vi "Dispense FN - ON - State Status (SubVI).vi"(0 "Values IN":T1 {"Drain Time (s)" format="%.2f"; "Drain Rate (g/sec)" format="%.2f"}, 7 "Min Spray Complete?":bool, 8 "Spray Count":i32, 9 "Measure Delay Complete?":bool, 11 "Max Spray Complete?":bool) -> (15 "Dispense Timeout?":bool, 17 "Complete":bool, 19 "OFF Signal":bool)   [LabVIEW 2009]
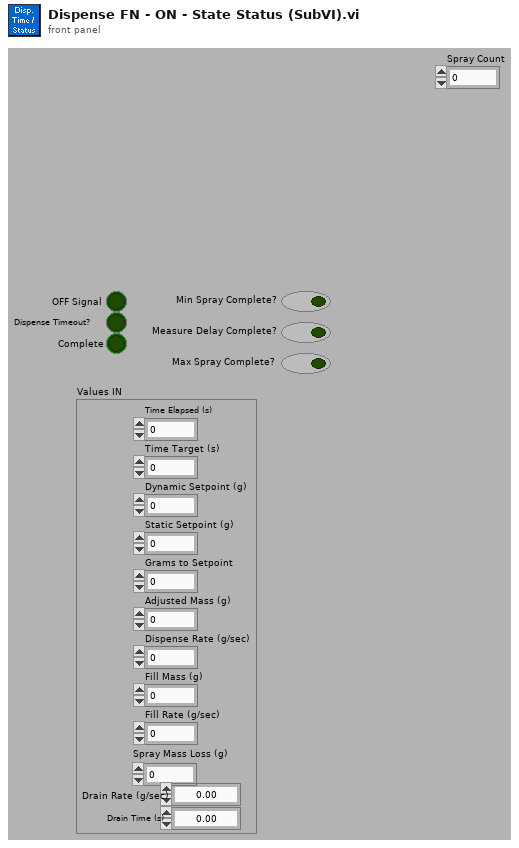
[diagram p1: front panel]
types:
  T1 = cluster{"Time Elapsed (s)":dbl, "Time Target (s)":dbl, "Dynamic Setpoint (g)":dbl, "Static Setpoint (g)":dbl, "Grams to Setpoint":dbl, "Adjusted Mass (g)":dbl, "Dispense Rate (g/sec)":dbl, "Fill Mass (g)":dbl, "Fill Rate (g/sec)":dbl, "Spray Mass Loss (g)":dbl, "Drain Rate (g/sec)":dbl, "Drain Time (s)":dbl}
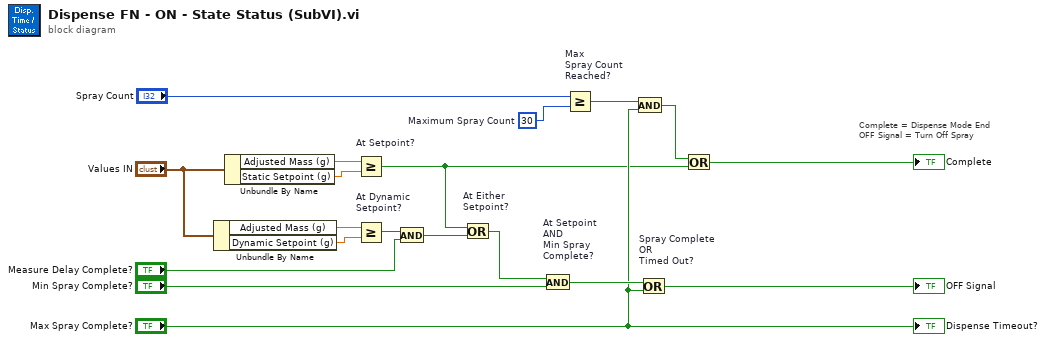
[diagram p0: block diagram]
diagram:
  w7 = 30  # Maximum Spray Count
  # "Complete = Dispense Mode End\nOFF Signal = Turn Off Spray"
  n1 = Unbundle By Name("Values IN") -> ("Adjusted Mass (g)"=w14:dbl, "Dynamic Setpoint (g)"=w15:dbl)
  n2 = Unbundle By Name("Values IN") -> ("Adjusted Mass (g)"=w18:dbl, "Static Setpoint (g)"=w17:dbl)
  n3 = Greater Or Equal? "At Setpoint?"(x=w18, y=w17) -> (x >= y?=w2:bool)
  n4 = Greater Or Equal? "At Dynamic\nSetpoint?"(x=w14, y=w15) -> (x >= y?=w19:bool)
  n5 = And(x=w19, y="Measure Delay Complete?") -> (x .and. y?=w11:bool)
  n6 = Or "At Either\nSetpoint?"(x=w2, y=w11) -> (x .or. y?=w10:bool)
  n7 = And "At Setpoint\nAND\nMin Spray\nComplete?"(x=w10, y="Min Spray Complete?") -> (x .and. y?=w9:bool)
  n8 = Greater Or Equal? "Max\nSpray Count\nReached?"(x="Spray Count", y=w7) -> (x >= y?=w6:bool)
  n9 = And(x=w6, y="Max Spray Complete?") -> (x .and. y?=w1:bool)
  n10 = Or "Spray Complete\nOR\nTimed Out?"(x=w9, y="Max Spray Complete?") -> (x .or. y?=→"OFF Signal":bool)
  n11 = Or(x=w1, y=w2) -> (x .or. y?=→"Complete":bool)
  "Dispense Timeout?" <- "Max Spray Complete?"
